vi "Read SmartRelay INI File.vi"(8 "error in":errorcluster, 11 "Path":path) -> (0 "error out":errorcluster, 2 "SmartRelay_Config Settings":T1, 3 "SmartRelay_Info":T2)   [LabVIEW 2018]
uses:
  <vilib>/ORNL/CSEISMIC DDS/CSEISMIC DDS Base/Data Types/SmartRelay_Info.ctl
  <vilib>/ORNL/CSEISMIC DDS/CSEISMIC DDS Base/Data Types/Controls/DeviceID.ctl
  Controls/Smart Relay Config Settings.ctl
  <vilib>/Utility/config.llb/Read Key (String).vi
  <vilib>/Utility/config.llb/Read Key (U32).vi
  <vilib>/Utility/config.llb/Read Key (Double).vi
  <vilib>/Utility/config.llb/NI_LVConfig.lvlib
  <vilib>/ORNL/CSEISMIC DDS/CSEISMIC DDS Base/CSEISMIC DDS.lvclass
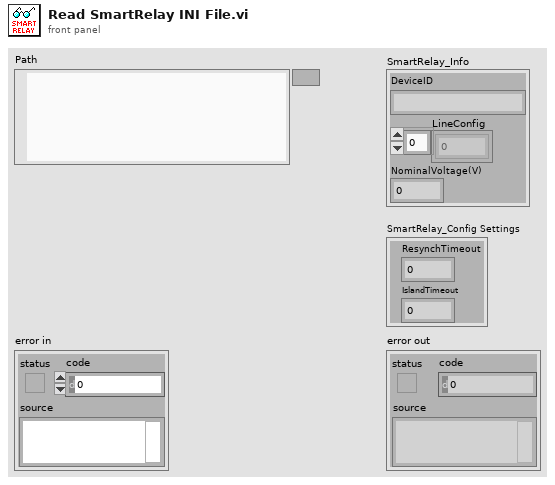
[diagram p1: front panel]
types:
  T1 = typedef "Smart Relay Config Settings.ctl" = cluster{"ResynchTimeout":dbl, "IslandTimeout":dbl}
  T2 = typedef "CSEISMIC DDS.lvlib/CSEISMIC DDS.lvclass/SmartRelay_Info.ctl" = cluster{"DeviceID":T3, "LineConfig":u8[], "NominalVoltage(V)":dbl}
  T3 = typedef "CSEISMIC DDS.lvlib/CSEISMIC DDS.lvclass/DeviceID.ctl" = string
  T4 = typedef "NI_LVConfig.lvlib/Config Data RefNum.ctl" = refnum<k1>
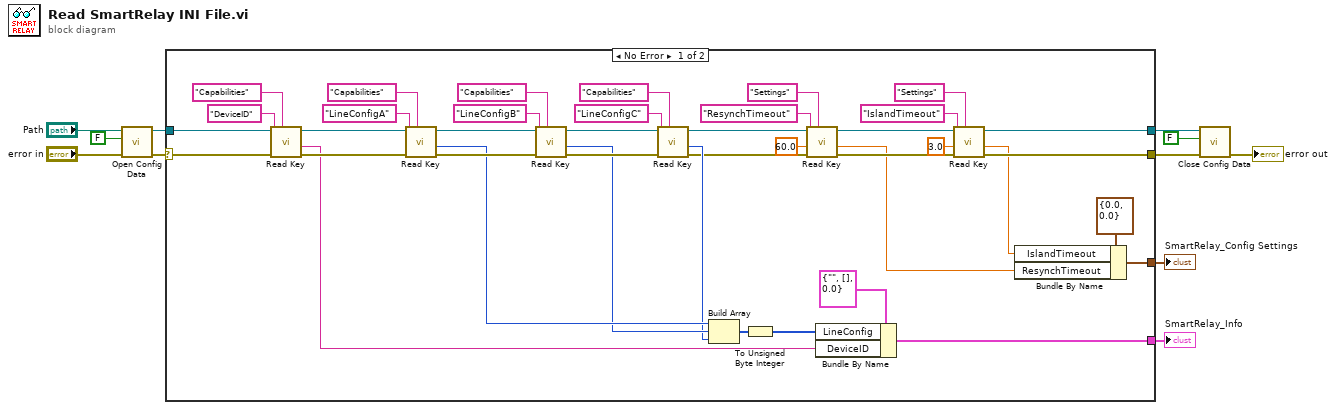
[diagram p0: block diagram]
diagram:
  n1 = call <vilib>:"Open Config Data.vi"("error in (no error)"="error in", "create file if necessary (T)"=FALSE, "configuration file path"="Path") -> ("error out"=w9:errorcluster, "refnum"=w8:T4)  [unwired: 6 in, 1 out]
  n2 = case shown="No Error" w9 {
    selector: w9 -> [w32 w52]
    tunnel: w8 -> [w33 w53]
    tunnel: [w18 w53] -> w7
    tunnel: [w17 w52] -> w6
    tunnel: [w29 _] -> w2
    tunnel: [w13 _] -> w1
    frame No Error {
      n3 = call-poly <vilib>:"Read Key.vi"("section"="Capabilities", "error in (no error)"=w32, "key"="DeviceID", "refnum"=w33) -> ("error out"=w35:errorcluster, "value"=w12:string, "refnum out"=w36:T4)  [unwired: 4 in, 1 out]
      n4 = call-poly <vilib>:"Read Key.vi"("section"="Capabilities", "error in (no error)"=w35, "key"="LineConfigA", "refnum"=w36) -> ("error out"=w44:errorcluster, "value"=w41:u32, "refnum out"=w45:T4)  [unwired: 4 in, 1 out]
      n5 = call-poly <vilib>:"Read Key.vi"("section"="Capabilities", "error in (no error)"=w44, "key"="LineConfigB", "refnum"=w45) -> ("error out"=w42:errorcluster, "value"=w40:u32, "refnum out"=w43:T4)  [unwired: 4 in, 1 out]
      n6 = call-poly <vilib>:"Read Key.vi"("section"="Capabilities", "error in (no error)"=w42, "key"="LineConfigC", "refnum"=w43) -> ("error out"=w25:errorcluster, "value"=w39:u32, "refnum out"=w26:T4)  [unwired: 4 in, 1 out]
      n7 = Build Array(w41, w40, w39) -> (w34:u32[])
      n8 = To Unsigned Byte Integer(number=w34) -> (unsigned 8bit integer=w30:u8[])
      n9 = call-poly <vilib>:"Read Key.vi"("section"="Settings", "error in (no error)"=w25, "default value"=60.0, "key"="ResynchTimeout", "refnum"=w26) -> ("error out"=w20:errorcluster, "value"=w14:dbl, "refnum out"=w19:T4)  [unwired: 3 in, 1 out]
      n10 = Bundle By Name(cluster=T2 {"DeviceID"="", "LineConfig"=[], "NominalVoltage(V)"=0.0} ("SmartRelay_Info"), "LineConfig"=w30, "DeviceID"=w12) -> (w29:T2)
      n11 = call-poly <vilib>:"Read Key.vi"("section"="Settings", "error in (no error)"=w20, "default value"=3.0, "key"="IslandTimeout", "refnum"=w19) -> ("error out"=w17:errorcluster, "value"=w15:dbl, "refnum out"=w18:T4)  [unwired: 3 in, 1 out]
      n12 = Bundle By Name(cluster=T1 {"ResynchTimeout"=0.0, "IslandTimeout"=0.0}, "IslandTimeout"=w15, "ResynchTimeout"=w14) -> (w13:T1)
    }
    frame Error {
    }
  }
  "SmartRelay_Info" <- w2
  "SmartRelay_Config Settings" <- w1
  n13 = call <vilib>:"Close Config Data.vi"("error in (no error)"=w6, "write file if changed (T)"=FALSE, "refnum"=w7) -> ("error out"=→"error out":errorcluster)  [unwired: 7 in, 1 out]
